vi "PrimaryInterfaceSendScript.vi"(8 "PrimaryInterface":refnum<k24>, 9 "script":string, 11 "error in":errorcluster) -> (3 "error out":errorcluster)   [LabVIEW 2020, in "UnderAutomation.UniversalRobots.lvlib"]
uses:
  UnderAutomation.UniversalRobots.lvlib
  C:/Users/fg/Documents/UniversalRobots.vi/LabVIEW_2024/UnderAutomation.UniversalRobots/lib/UnderAutomation.UniversalRobots.dll
  LabVIEW_2024/UnderAutomation.UniversalRobots/lib/UnderAutomation.UniversalRobots.dll
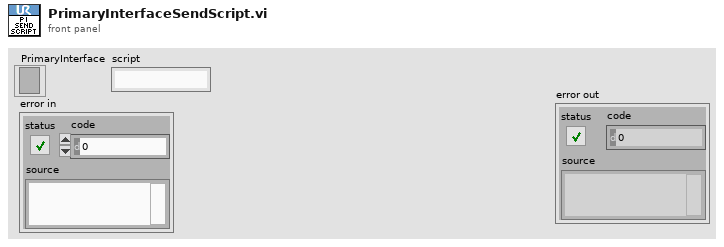
[diagram p1: front panel]
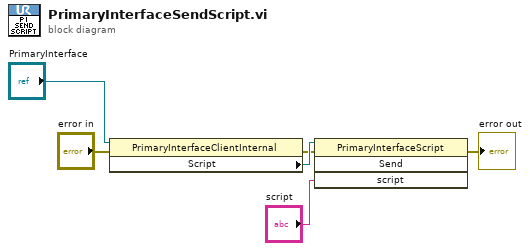
[diagram p0: block diagram]
diagram:
  n1 = property class="PrimaryInterfaceClientInternal"(reference="PrimaryInterface", error in="error in") -> (error out=w1:errorcluster, "Script"=w4:refnum<k24>)  [unwired: 1 out]
  n2 = invoke class="PrimaryInterfaceScript" method="Send"(reference=w4, error in=w1, "script"="script") -> (error out=→"error out":errorcluster)  [unwired: 1 in, 3 out]
